vi "Discover Nodes.vi"(8 "error in":errorcluster, 11 "Interactor in":refnum<class "Interactor.lvclass">) -> (0 "error out":errorcluster, 3 "Interactor out":refnum<class "Interactor.lvclass">)   [LabVIEW 2024, in "Interactor.lvlib" / "Interactor.lvclass"]
uses:
  Interactor.lvclass
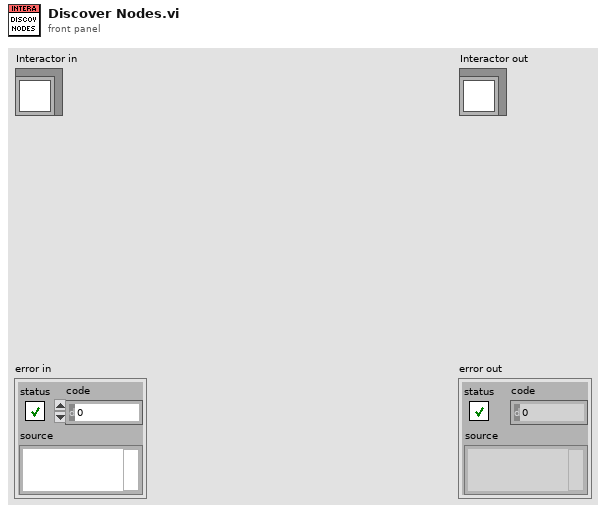
[diagram p1: front panel]
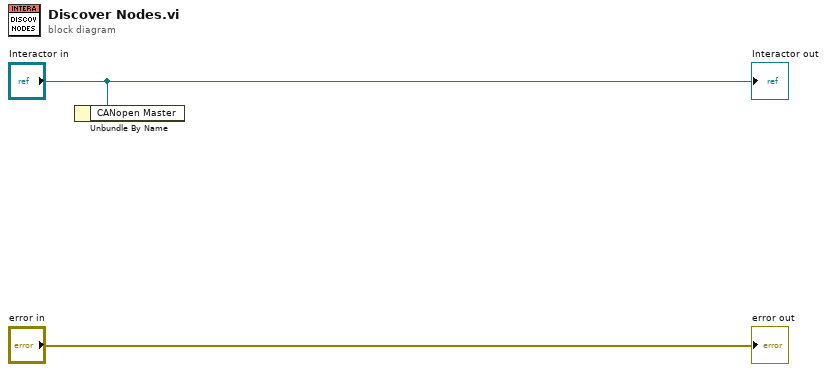
[diagram p0: block diagram]
diagram:
  n1 = Unbundle By Name("Interactor in") -> ()  [unwired: 1 out]
  "error out" <- "error in"
  "Interactor out" <- "Interactor in"
